vi "Untitled 1.vi"() -> ()   [LabVIEW 2014]
uses:
  Drying Macine 07.07.2015/Master/Masterv2.lvclass
panel:
  out "User Enable":bool
  out "Admin Enable":bool
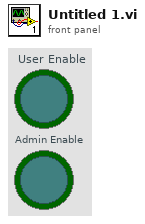
[diagram p1: front panel]
types:
  T1 = enum16{"9", "8", "7", "6", "5", "4", "3", "2", "1", "0"}[]
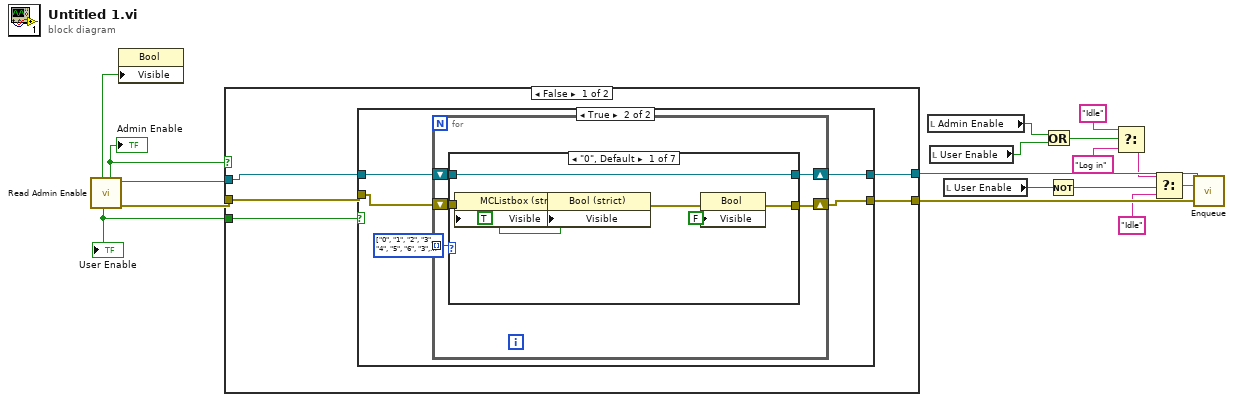
[diagram p0: block diagram]
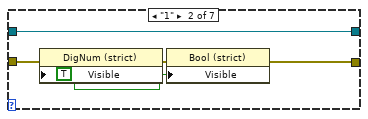
[diagram p3: hidden frame]
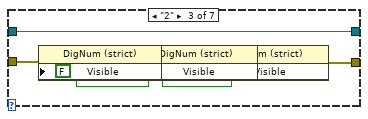
[diagram p4: hidden frame]
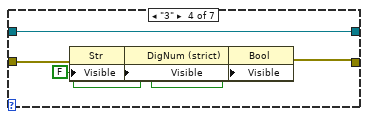
[diagram p5: hidden frame]
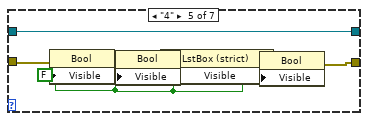
[diagram p6: hidden frame]
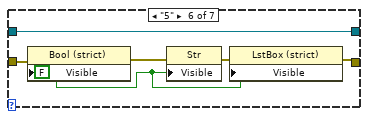
[diagram p7: hidden frame]
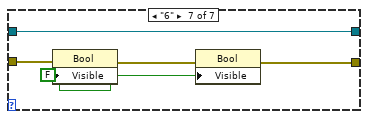
[diagram p8: hidden frame]
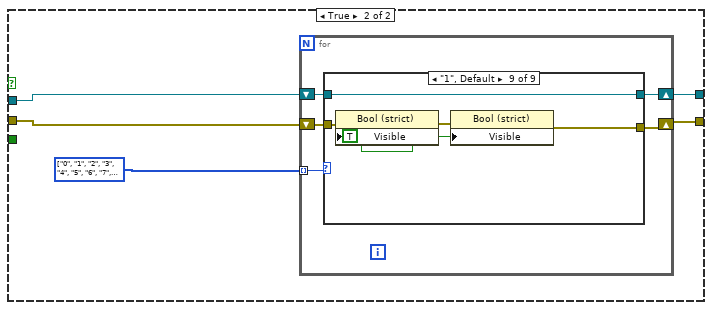
[diagram p9: hidden frame]
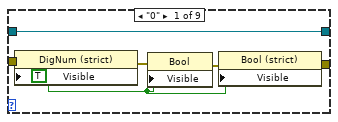
[diagram p10: hidden frame]
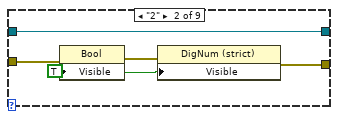
[diagram p11: hidden frame]
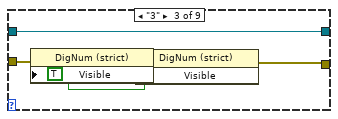
[diagram p12: hidden frame]
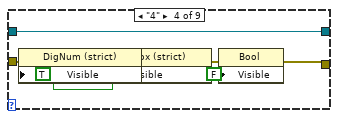
[diagram p13: hidden frame]
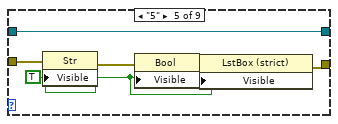
[diagram p14: hidden frame]
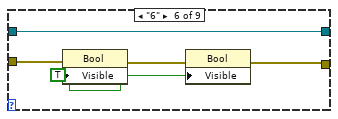
[diagram p15: hidden frame]
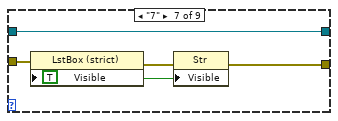
[diagram p16: hidden frame]
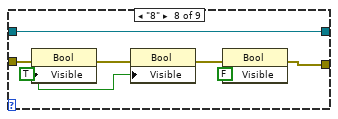
[diagram p17: hidden frame]
diagram:
  n1 = call-dynamic "Read Admin Enable.vi"() -> ("error out"=w14:errorcluster, "Masterv2 out"=w15:refnum<class "Masterv2.lvclass">, "Admin Enable"=w5:bool, "User Enable"=w4:bool, "Programmer Enable"=w13:bool)  [unwired: 6 in, 1 out]
  "Admin Enable" <- w5
  "User Enable" <- w4
  n2 = property on="Property Node" class="Bool"("Visible"=w13) -> ()  [unwired: 2 in, 2 out]
  n3 = case shown="False" w5 {
    tunnel: w4 -> [w22 _]
    tunnel: w14 -> [w20 w81]
    tunnel: w15 -> [w21 w79]
    tunnel: [w18 w80] -> w16
    tunnel: [w19 w78] -> w17
    frame False {
      n4 = case shown="True" w22 {
        tunnel: w21 -> [w24 w29]
        tunnel: w20 -> [w23 w28]
        tunnel: [w24 w27] -> w19
        tunnel: [w23 w26] -> w18
        frame False {
        }
        frame True {
          w25 = enum16{"6", "5", "4", "3", "2", "1", "0"}[] [enum."0", enum."1", enum."2", enum."3", enum."4", enum."5", enum."6", enum."3", enum."4", enum."5", enum."6"] items=["6", "5", "4", "3", "2", "1", "0"]
          n5 = for {
            shift-right: [w32] -> w27
            shift-left: w29 -> [w33]
            shift-right: [w30] -> w26
            shift-left: w28 -> [w34]
            tunnel: w25 -> [w31] mode=indexing
            n6 = case shown="\"0\", Default" w31 {
              tunnel: w34 -> [w40 w45 w51 w57 w62 w70 w75]
              tunnel: w33 -> [w41 w46 w52 w58 w65 w71 w76]
              tunnel: [w41 w46 w52 w58 w65 w71 w76] -> w32
              tunnel: [w37 w43 w48 w54 w60 w67 w73] -> w30
              frame "0", Default {
                w36 = TRUE ("Visible")
                n7 = property on="Property Node" class="MCListbox (strict)"(error in=w40, "Visible"=w36) -> (error out=w39:errorcluster)  [unwired: 1 in, 1 out]
                n8 = property on="Property Node" class="Bool (strict)"(error in=w39, "Visible"=w36) -> (error out=w38:errorcluster)  [unwired: 1 in, 1 out]
                n9 = property on="Property Node" class="Bool"(error in=w38, "Visible"=FALSE) -> (error out=w37:errorcluster)  [unwired: 1 in, 1 out]
              }
              frame "1" {
                w42 = TRUE ("Visible")
                n10 = property on="Property Node" class="DigNum (strict)"(error in=w45, "Visible"=w42) -> (error out=w44:errorcluster)  [unwired: 1 in, 1 out]
                n11 = property on="Property Node" class="Bool (strict)"(error in=w44, "Visible"=w42) -> (error out=w43:errorcluster)  [unwired: 1 in, 1 out]
              }
              frame "2" {
                w47 = FALSE ("Visible")
                n12 = property on="Property Node" class="DigNum (strict)"(error in=w51, "Visible"=w47) -> (error out=w50:errorcluster)  [unwired: 1 in, 1 out]
                n13 = property on="Property Node" class="DigNum (strict)"(error in=w50, "Visible"=w47) -> (error out=w49:errorcluster)  [unwired: 1 in, 1 out]
                n14 = property on="Property Node" class="DigNum (strict)"(error in=w49, "Visible"=w47) -> (error out=w48:errorcluster)  [unwired: 1 in, 1 out]
              }
              frame "3" {
                w53 = FALSE ("Visible")
                n15 = property on="Property Node" class="Str"(error in=w57, "Visible"=w53) -> (error out=w56:errorcluster)  [unwired: 1 in, 1 out]
                n16 = property on="Property Node" class="DigNum (strict)"(error in=w56, "Visible"=w53) -> (error out=w55:errorcluster)  [unwired: 1 in, 1 out]
                n17 = property on="Property Node" class="Bool"(error in=w55, "Visible"=w53) -> (error out=w54:errorcluster)  [unwired: 1 in, 1 out]
              }
              frame "4" {
                w59 = FALSE ("Visible")
                n18 = property on="Property Node" class="Bool"(error in=w62, "Visible"=w59) -> (error out=w63:errorcluster)  [unwired: 1 in, 1 out]
                n19 = property on="Property Node" class="Bool"(error in=w63, "Visible"=w59) -> (error out=w64:errorcluster)  [unwired: 1 in, 1 out]
                n20 = property on="Property Node" class="LstBox (strict)"(error in=w64, "Visible"=w59) -> (error out=w61:errorcluster)  [unwired: 1 in, 1 out]
                n21 = property on="Property Node" class="Bool"(error in=w61, "Visible"=w59) -> (error out=w60:errorcluster)  [unwired: 1 in, 1 out]
              }
              frame "5" {
                w66 = FALSE ("Visible")
                n22 = property on="Property Node" class="Bool (strict)"(error in=w70, "Visible"=w66) -> (error out=w69:errorcluster)  [unwired: 1 in, 1 out]
                n23 = property on="Property Node" class="Str"(error in=w69, "Visible"=w66) -> (error out=w68:errorcluster)  [unwired: 1 in, 1 out]
                n24 = property on="Property Node" class="LstBox (strict)"(error in=w68, "Visible"=w66) -> (error out=w67:errorcluster)  [unwired: 1 in, 1 out]
              }
              frame "6" {
                w72 = FALSE ("Visible")
                n25 = property on="Property Node" class="Bool"(error in=w75, "Visible"=w72) -> (error out=w74:errorcluster)  [unwired: 1 in, 1 out]
                n26 = property on="Property Node" class="Bool"(error in=w74, "Visible"=w72) -> (error out=w73:errorcluster)  [unwired: 1 in, 1 out]
              }
            }
          }
        }
      }
    }
    frame True {
      w77 = T1 [enum."0", enum."1", enum."2", enum."3", enum."4", enum."5", enum."6", enum."7", enum."8", enum."9"] items=["9", "8", "7", "6", "5", "4", "3", "2", "1", "0"]
      n27 = for {
        shift-right: [w84] -> w78
        shift-left: w79 -> [w85]
        shift-right: [w82] -> w80
        shift-left: w81 -> [w86]
        tunnel: w77 -> [w83] mode=indexing
        n28 = case shown="\"1\", Default" w83 {
          tunnel: w86 -> [w91 w96 w101 w108 w114 w119 w124 w131 w136]
          tunnel: w85 -> [w92 w97 w102 w109 w115 w120 w125 w132 w137]
          tunnel: [w92 w97 w102 w109 w115 w120 w125 w132 w137] -> w84
          tunnel: [w88 w94 w99 w105 w110 w117 w122 w128 w134] -> w82
          frame "0" {
            w87 = TRUE ("Visible")
            n29 = property on="Property Node" class="DigNum (strict)"(error in=w91, "Visible"=w87) -> (error out=w90:errorcluster)  [unwired: 1 in, 1 out]
            n30 = property on="Property Node" class="Bool"(error in=w90, "Visible"=w87) -> (error out=w89:errorcluster)  [unwired: 1 in, 1 out]
            n31 = property on="Property Node" class="Bool (strict)"(error in=w89, "Visible"=w87) -> (error out=w88:errorcluster)  [unwired: 1 in, 1 out]
          }
          frame "2" {
            w93 = TRUE ("Visible")
            n32 = property on="Property Node" class="Bool"(error in=w96, "Visible"=w93) -> (error out=w95:errorcluster)  [unwired: 1 in, 1 out]
            n33 = property on="Property Node" class="DigNum (strict)"(error in=w95, "Visible"=w93) -> (error out=w94:errorcluster)  [unwired: 1 in, 1 out]
          }
          frame "3" {
            w98 = TRUE ("Visible")
            n34 = property on="Property Node" class="DigNum (strict)"(error in=w101, "Visible"=w98) -> (error out=w100:errorcluster)  [unwired: 1 in, 1 out]
            n35 = property on="Property Node" class="DigNum (strict)"(error in=w100, "Visible"=w98) -> (error out=w99:errorcluster)  [unwired: 1 in, 1 out]
          }
          frame "4" {
            w104 = TRUE ("Visible")
            n36 = property on="Property Node" class="DigNum (strict)"(error in=w108, "Visible"=w104) -> (error out=w107:errorcluster)  [unwired: 1 in, 1 out]
            n37 = property on="Property Node" class="MCListbox (strict)"(error in=w107, "Visible"=w104) -> (error out=w106:errorcluster)  [unwired: 1 in, 1 out]
            n38 = property on="Property Node" class="Bool"(error in=w106, "Visible"=FALSE) -> (error out=w105:errorcluster)  [unwired: 1 in, 1 out]
          }
          frame "5" {
            w111 = TRUE ("Visible")
            n39 = property on="Property Node" class="Str"(error in=w114, "Visible"=w111) -> (error out=w113:errorcluster)  [unwired: 1 in, 1 out]
            n40 = property on="Property Node" class="Bool"(error in=w113, "Visible"=w111) -> (error out=w112:errorcluster)  [unwired: 1 in, 1 out]
            n41 = property on="Property Node" class="LstBox (strict)"(error in=w112, "Visible"=w111) -> (error out=w110:errorcluster)  [unwired: 1 in, 1 out]
          }
          frame "6" {
            w116 = TRUE ("Visible")
            n42 = property on="Property Node" class="Bool"(error in=w119, "Visible"=w116) -> (error out=w118:errorcluster)  [unwired: 1 in, 1 out]
            n43 = property on="Property Node" class="Bool"(error in=w118, "Visible"=w116) -> (error out=w117:errorcluster)  [unwired: 1 in, 1 out]
          }
          frame "7" {
            w121 = TRUE ("Visible")
            n44 = property on="Property Node" class="LstBox (strict)"(error in=w124, "Visible"=w121) -> (error out=w123:errorcluster)  [unwired: 1 in, 1 out]
            n45 = property on="Property Node" class="Str"(error in=w123, "Visible"=w121) -> (error out=w122:errorcluster)  [unwired: 1 in, 1 out]
          }
          frame "8" {
            w127 = TRUE ("Visible")
            n46 = property on="Property Node" class="Bool"(error in=w131, "Visible"=w127) -> (error out=w130:errorcluster)  [unwired: 1 in, 1 out]
            n47 = property on="Property Node" class="Bool"(error in=w130, "Visible"=w127) -> (error out=w129:errorcluster)  [unwired: 1 in, 1 out]
            n48 = property on="Property Node" class="Bool"(error in=w129, "Visible"=FALSE) -> (error out=w128:errorcluster)  [unwired: 1 in, 1 out]
          }
          frame "1", Default {
            w133 = TRUE ("Visible")
            n49 = property on="Property Node" class="Bool (strict)"(error in=w136, "Visible"=w133) -> (error out=w135:errorcluster)  [unwired: 1 in, 1 out]
            n50 = property on="Property Node" class="Bool (strict)"(error in=w135, "Visible"=w133) -> (error out=w134:errorcluster)  [unwired: 1 in, 1 out]
          }
        }
      }
    }
  }
  n51 = local read "Admin Enable"() -> (w3:bool)
  n52 = local read "User Enable"() -> (w2:bool)
  n53 = local read "User Enable"() -> (w1:bool)
  n54 = Or(x=w3, y=w2) -> (x .or. y?=w10:bool)
  n55 = Not(x=w1) -> (.not. x?=w8:bool)
  n56 = Select(t="Idle", s=w10, f="Log in" ("State")) -> (s? t:f=w9:string)
  n57 = Select(t=w9, s=w8, f="Idle") -> (s? t:f=w6:string)
  n58 = call-dynamic "Enqueue.vi"("error in (no error)"=w16, "State"=w6, "Masterv2 in"=w17) -> ()  [unwired: 7 in, 2 out]
